vi "Create Object.vi"(11 "jettl Event Actor in":refnum<class "jettl Event Actor.lvclass">) -> (2 "jettl Event Actor":refnum<class "jettl Event Actor.lvclass">)   [LabVIEW 2021, in "jettl.lvlib" / "jettl Event Actor.lvlib" / "jettl Event Actor.lvclass"]
uses:
  jettl Event Actor.lvclass
  jettl.lvlib
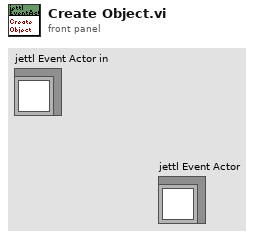
[diagram p1: front panel]
types:
  T1 = cluster{"Caller Queue Alias":string, "Caller Msg Queue DVR":refnum<data-value>, "Self Event Alias":string, "Self Msg Event DVR":refnum<data-value>, "Error":errorcluster}
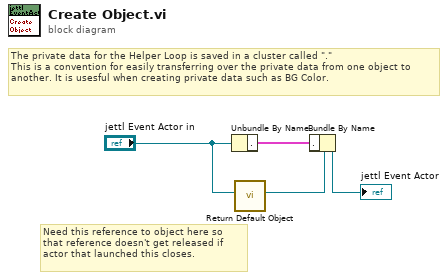
[diagram p0: block diagram]
diagram:
  # "The private data for the Helper Loop is saved in a cluster called \".\"\nThis is a convention for easily transferring over the private data from one object to another. It is usesful when creating private data such as BG Color."
  # "Need this reference to object here so that reference doesn't get released if actor that launched this closes."
  n1 = Unbundle By Name("jettl Event Actor in") -> ("."=w4:T1)
  n2 = call "Return Default Object.vi"("Object"="jettl Event Actor in") -> ("Default Object Instance"=w3:refnum<class "jettl Event Actor.lvclass">)  [unwired: 10 in]
  n3 = Bundle By Name(cluster=w3, "."=w4) -> (→"jettl Event Actor":refnum<class "jettl Event Actor.lvclass">)
